vi "Extract Numbers2.vi"(4 "String":string="Counting to five:\none 2 three 4.0 five") -> (0 "After Number":string, 1 "Output Array":dbl[](array[numeric]) format="%0.2f", 2 "Output Digit":dbl)   [LabVIEW 2014]
doc: "Finds all numbers in the given string and puts them into an array as double-precision numbers. All of the following formats are recognized:\n123 1.23 .123 0.123 -1.23\nNo spaces or other characters may appear within the number, but any characters may appear before or after the number.\nThis example assumes that the input string contains periods and not commas for the decimal separator."
panel:
  out "Output Strings":string[](array[string])
  # "Enter a sentence in the string control and press the run\narrow to execute the VI.  All of the numbers in the string \nwill be placed in the array below.  Please note that \nnumbers that are spelled out (\"one\") are not interpreted \nas numbers.  Scientific notation is not handled by this\nexample.  Press <ctrl-h> for more information."
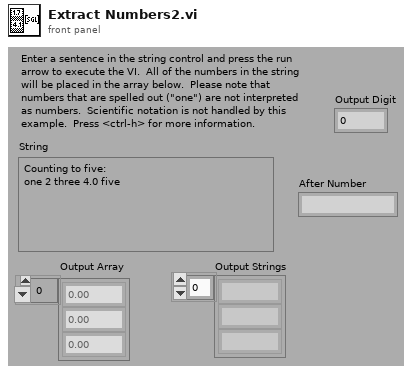
[diagram p1: front panel]
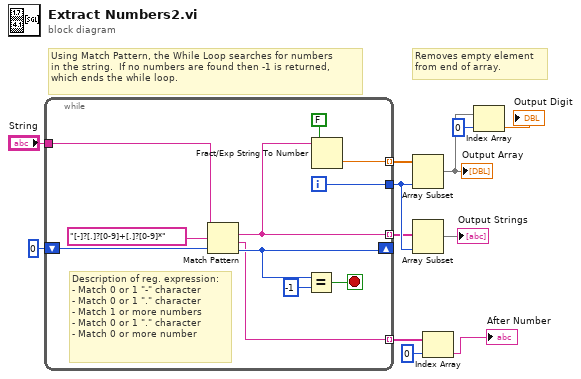
[diagram p0: block diagram]
diagram:
  # "Removes empty element\nfrom end of array."
  # "Using Match Pattern, the While Loop searches for numbers\nin the string.  If no numbers are found then -1 is returned,\nwhich ends the while loop."
  n1 = while {
    tunnel: "String" -> [w21]
    tunnel: [w23] -> w9
    shift-left: 0 -> [w17]
    shift-right: [w16] -> _
    tunnel: [w20] -> w10 mode=indexing
    tunnel: [w14] -> w8 mode=indexing
    tunnel: [w13] -> w6 mode=indexing
    i -> [w23]
    stop <- w19 stop-if-true
    # "Description of reg. expression:\n- Match 0 or 1 \"-\" character\n- Match 0 or 1 \".\" character\n- Match 1 or more numbers\n- Match 0 or 1 \".\" character\n- Match 0 or more number"
    n2 = Match Pattern(string=w21, regular expression="[-]?[.]?[0-9]+[.]?[0-9]*", offset (0)=w17) -> (match substring=w14:string, after substring=w13:string, offset past match=w16:i32)  [unwired: 1 out]
    n3 = Equal?(x=w16, y=-1) -> (x = y?=w19:bool)
    n4 = Fract/Exp String To Number(use system decimal point (T)=FALSE, string=w14) -> (number=w20:dbl)  [unwired: 3 out]
  }
  n5 = Array Subset(array=w10, length=w9) -> (w3:dbl[])  [unwired: 1 in]
  "Output Array" <- w3
  n6 = Array Subset(array=w8, length=w9) -> (→"Output Strings":string[])  [unwired: 1 in]
  n7 = Index Array(array=w6, index=0) -> (element=→"After Number":string)
  n8 = Index Array(array=w3, index=0) -> (element=→"Output Digit":dbl)
